vi "AVI Video-Get refs.vi"(8 "error in (no error)":errorcluster) -> (0 "error out":errorcluster, 2 "AVI mode":T5, 3 "Frame Size":u32, 4 "Green PMT is ON":bool, 5 "Red AVI":T1, 6 "Green AVI":T1, 7 "Red PMT is ON":bool)   [LabVIEW 2013]
uses:
  Typedefs/AVI implementation enum.ctl
  Typedefs/AVI Refs cluster.ctl
  <vilib>/vision/Avi.llb/IMAQ AVI2 Refnum.ctl
  <vilib>/vision/Image Controls.llb/IMAQ Image.ctl
  <vilib>/vision/Avi1.llb/AviRefnum.ctl
  Global Variables/General Globals.vi
panel:
  # "SUBROUTINE VI"
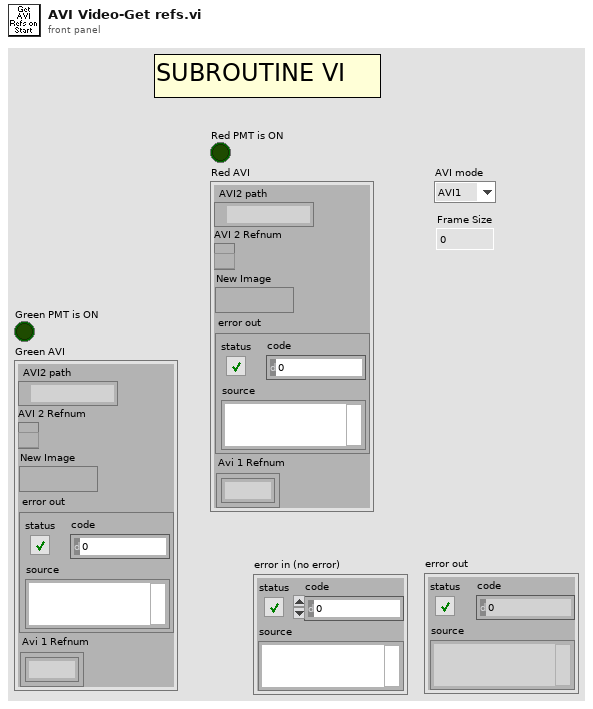
[diagram p1: front panel]
types:
  T1 = typedef "AVI Refs cluster.ctl" = cluster{"AVI2 path":path, "AVI 2 Refnum":T2, "New Image":T3, "error out":errorcluster, "Avi 1 Refnum":T4}
  T2 = typedef "IMAQ AVI2 Refnum.ctl" = refnum<k20>
  T3 = typedef "IMAQ Image.ctl" = refnum<image>
  T4 = typedef "AviRefnum.ctl" = refnum<k1>
  T5 = typedef "AVI implementation enum.ctl" = enum16{"AVI1", "AVI2"}
  T6 = typedef "Frame Size.ctl" = u16
  T7 = cluster{"AVI mode":T5, "Red AVI":T1, bool, "Green AVI":T1, bool, "Frame Size":T6}
  T8 = typedef "AOL_Globals.ctl" = cluster{"Imaging Protocol":T9, "Number of POI":u16, "Number of Miniscans":u16, "Number of Trials":u16, "Number of Cycles ":u64, "# Averaged Frames":u16, "Laser power (%)":u8, "Pockels":dbl, "Acquisition Length (sec)":dbl, "Fill time (us)":dbl, "POI Dwell time (us)":dbl, "Miniscan Dwell time per pixel (us)":dbl, "PMT 1":dbl, "PMT 2":dbl, "Back Apperture":dbl, "Frame Size":T6, "Center Frequency":dbl, "Field of View":dbl, "DwellTime (us)":dbl, "Wavelength (nm)":dbl, "Zoom":dbl, "AOL Z":dbl, "AOL Mode":T10, "GridXY":dbl, "GridZ":dbl, "TriggerPeriod (sec)":dbl, "Number of Pixels in Miniscan":u16, "Experiment folder path":path, "X centre":dbl, "Y centre":dbl, "Angle (degrees)":dbl, "Plane Mode":T11, "Threshold":u16[], "Regenerate Chirps":bool, "Rectangle ROI length (pixels)":u16, "Rectangle ROI height (pixels)":u16, "AOD fill":u16, "Samples Wait after Trigger":u16, "StartUp Delay":i32, "Slip Cycle":u32, "Add Cycle":bool}
  T9 = typedef "Imaging Protocols enum.ctl" = enum16{"AOL Z-Stack", "Motor Z Stack", "Functional Acquisition", "Single Plane Acquisition", "Volume Acquisition", "Live Imaging", "Live Plane Imaging", "Live Volume Imaging"}
  T10 = typedef "AOL modes.ctl" = enum16{"Raster", "Structural", "Pointing", "Mini Scan", "Alignment"}
  T11 = typedef "Plane Mode.ctl" = u16
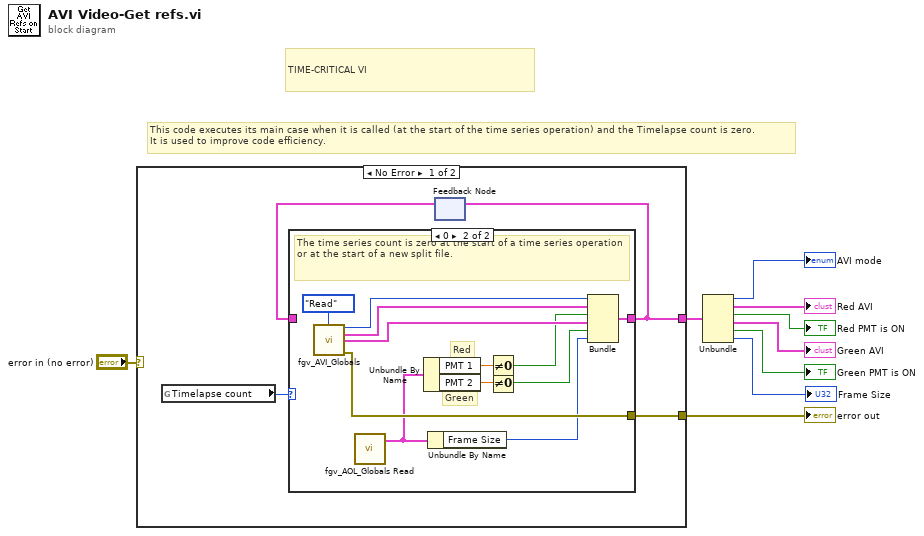
[diagram p0: block diagram]
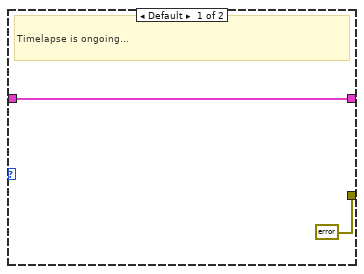
[diagram p2: hidden frame]
diagram:
  # "TIME-CRITICAL VI"
  # "This code executes its main case when it is called (at the start of the time series operation) and the Timelapse count is zero.\nIt is used to improve code efficiency."
  n1 = case shown="No Error" "error in (no error)" {
    selector: "error in (no error)" -> [_ w28]
    tunnel: [w13 _] -> w4
    tunnel: [w10 w28] -> w2
    frame No Error {
      n2 = global read "General Globals.vi" "Timelapse count"() -> (w11:u32)
      n3 = feedback #1() -> (w12:T7)  [unwired: 1 in]
      n4 = case shown="0" w11 {
        tunnel: [w15 w23] -> w13
        tunnel: w12 -> [w15 _]
        tunnel: [errorcluster {"status"=FALSE, "code"=0, "source"=""} ("error out") w22] -> w10
        frame Default {
          # "Timelapse is ongoing..."
        }
        frame 0 {
          # "Green"
          # "Red"
          # "The time series count is zero at the start of a time series operation or at the start of a new split file."
          n5 = call "fgv_AVI_Globals.vi"("Function"=enum16{"Intialize", "Write", "Read", "Clear"}."Read") -> ("AVI mode"=w26:T5, "Red AVI"=w25:T1, "Green AVI"=w24:T1, "error out"=w22:errorcluster)  [unwired: 11 in]
          n6 = call "fgv_AOL_Globals Read.vi"() -> ("AOL_Globals"=w18:T8)  [unwired: 9 in, 2 out]
          n7 = Unbundle By Name(w18) -> ("PMT 1"=w17:dbl, "PMT 2"=w16:dbl)
          n8 = Unbundle By Name(w18) -> ("Frame Size"=w21:T6)
          n9 = Not Equal To 0?(x=w17) -> (x != 0?=w20:bool)
          n10 = Not Equal To 0?(x=w16) -> (x != 0?=w19:bool)
          n11 = Bundle("AVI mode"=w26, "Red AVI"=w25, w20, "Green AVI"=w24, w19, "Frame Size"=w21) -> (w23:T7)  [unwired: 1 in]
        }
      }
      n12 = feedback-in #1(w13) -> ()
    }
    frame Error {
    }
  }
  "error out" <- w2
  n13 = Unbundle(w4) -> ("AVI mode"=→"AVI mode":T5, "Red AVI"=→"Red AVI":T1, →"Red PMT is ON":bool, "Green AVI"=→"Green AVI":T1, →"Green PMT is ON":bool, "Frame Size"=→"Frame Size":T6)
